vi "init.vi"(11 "Camera Idx":i32=1) -> (1 "Event Registration Refnum":refnum<event-registration>, 2 "htoupcam":i32, 3 "Cluster":cluster{"pWidth":i32, "pHeight":i32})   [LabVIEW 2016]
uses:
  Downloads/toupcamsdk/win/extras/labview/labviewdemo/toupcam.dll
  Downloads/toupcamsdk/win/extras/labview/labviewdemo/toupcam_labview.dll
panel:
  in  "Width":i32
  in  "Height":i32
  in  "Live Resolution":u16(ring) items=["1280*1024", "640*512", "320*256"]
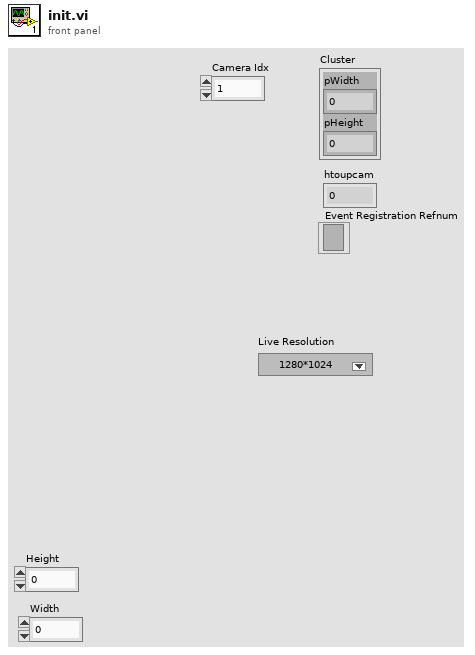
[diagram p1: front panel]
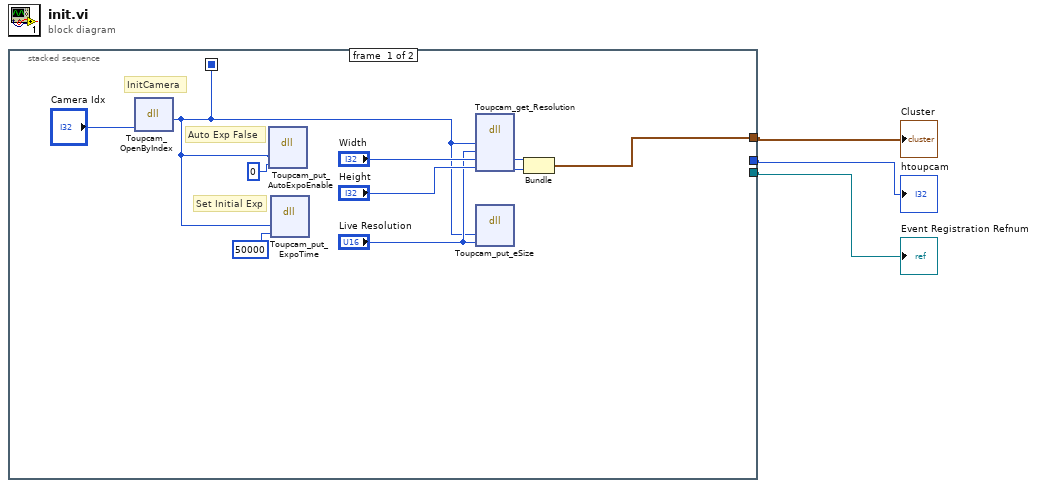
[diagram p0: block diagram]
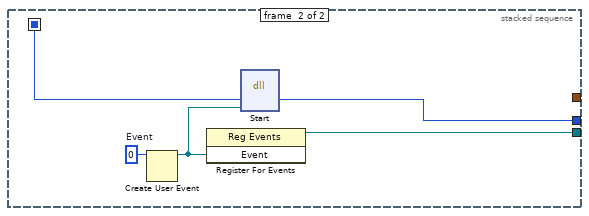
[diagram p2: hidden frame]
diagram:
  n1 = stacked-sequence {
    seq-local: [w5 _] -> [_ w15]
    tunnel: [_ w14] -> w1
    tunnel: [_ w16] -> w2
    tunnel: [w6 _] -> w3
    frame #0 {
      # "Auto Exp False"
      # "Set Initial Exp"
      # "InitCamera"
      n2 = dll-call lib="C:/Users/Thomassons/Downloads/toupcamsdk/win/extras/labview/labviewdemo/toupcam.dll" fn="Toupcam_OpenByIndex"("Index"="Camera Idx") -> ("return type"=w5:i32)  [unwired: 4 in, 2 out]
      n3 = dll-call lib="C:/Users/Thomassons/Downloads/toupcamsdk/win/extras/labview/labviewdemo/toupcam.dll" fn="Toupcam_put_AutoExpoEnable"("HToupcam"=w5, "bAutoExposure"=0) -> ()  [unwired: 6 in, 2 out]
      n4 = dll-call lib="C:/Users/Thomassons/Downloads/toupcamsdk/win/extras/labview/labviewdemo/toupcam.dll" fn="Toupcam_put_ExpoTime"("htoupcam"=w5, "Time"=50000) -> ()  [unwired: 6 in, 2 out]
      n5 = dll-call lib="C:/Users/Thomassons/Downloads/toupcamsdk/win/extras/labview/labviewdemo/toupcam.dll" fn="Toupcam_get_Resolution"("htoupcam"=w5, "ResNum"="Live Resolution", "pWidth"="Width", "pHeight"="Height") -> ("pWidth"=w11:i32, "pHeight"=w10:i32)  [unwired: 6 in, 2 out]
      n6 = dll-call lib="C:/Users/Thomassons/Downloads/toupcamsdk/win/extras/labview/labviewdemo/toupcam.dll" fn="Toupcam_put_eSize"("htoupcam"=w5, "nResolutionIndex"="Live Resolution") -> ()  [unwired: 6 in, 2 out]
      n7 = Bundle("pWidth"=w11, "pHeight"=w10) -> (w6:cluster{"pWidth":i32, "pHeight":i32})  [unwired: 1 in]
    }
    frame #1 {
      w17 = u32 0  # Event
      n8 = Create User Event(user event datatype=w17) -> (user event=w18:refnum<user-event>)  [unwired: 1 in, 1 out]
      n9 = register-events(w18) -> (reference out=w14:refnum<event-registration>)  [unwired: 2 in, 1 out]
      n10 = dll-call lib="C:/Users/Thomassons/Downloads/toupcamsdk/win/extras/labview/labviewdemo/toupcam_labview.dll" fn="Start"("htoupcam"=w15, "rwer"=w18) -> ("htoupcam"=w16:i32)  [unwired: 5 in, 2 out]
    }
  }
  "Cluster" <- w3
  "htoupcam" <- w2
  "Event Registration Refnum" <- w1
